vi "Maths.vi"(6 "Curseur tracé":i32, 8 "Indice curseur 2":i32, 9 "Indice curseur 1":i32, 10 "Graphe":T1(graph)) -> (0 "standard deviation":dbl caption="écart-type" format="%0.2f", 1 "valeur max":dbl, 2 "valeur min":dbl, 3 "mean":dbl caption="moyenne" format="%0.2f")   [LabVIEW 2013]
uses:
  <vilib>/Analysis/8numeric.llb/1D Numeric Integration.vi
  <vilib>/Analysis/NI_AALBase.lvlib
  <vilib>/Analysis/NI_AALPro.lvlib
panel:
  out "residue 2":dbl caption="résidu"
  out "offset":dbl
  out "damping":dbl caption="atténuation"
  out "amplitude":dbl
  out "R-square":dbl caption="R carré"
  out "residue":dbl caption="résidu"
  out "intercept":dbl caption="interception"
  out "slope":dbl caption="pente"
  out "Intégrale":dbl format="%0.4f"
  out "variance":dbl format="%0.2f"
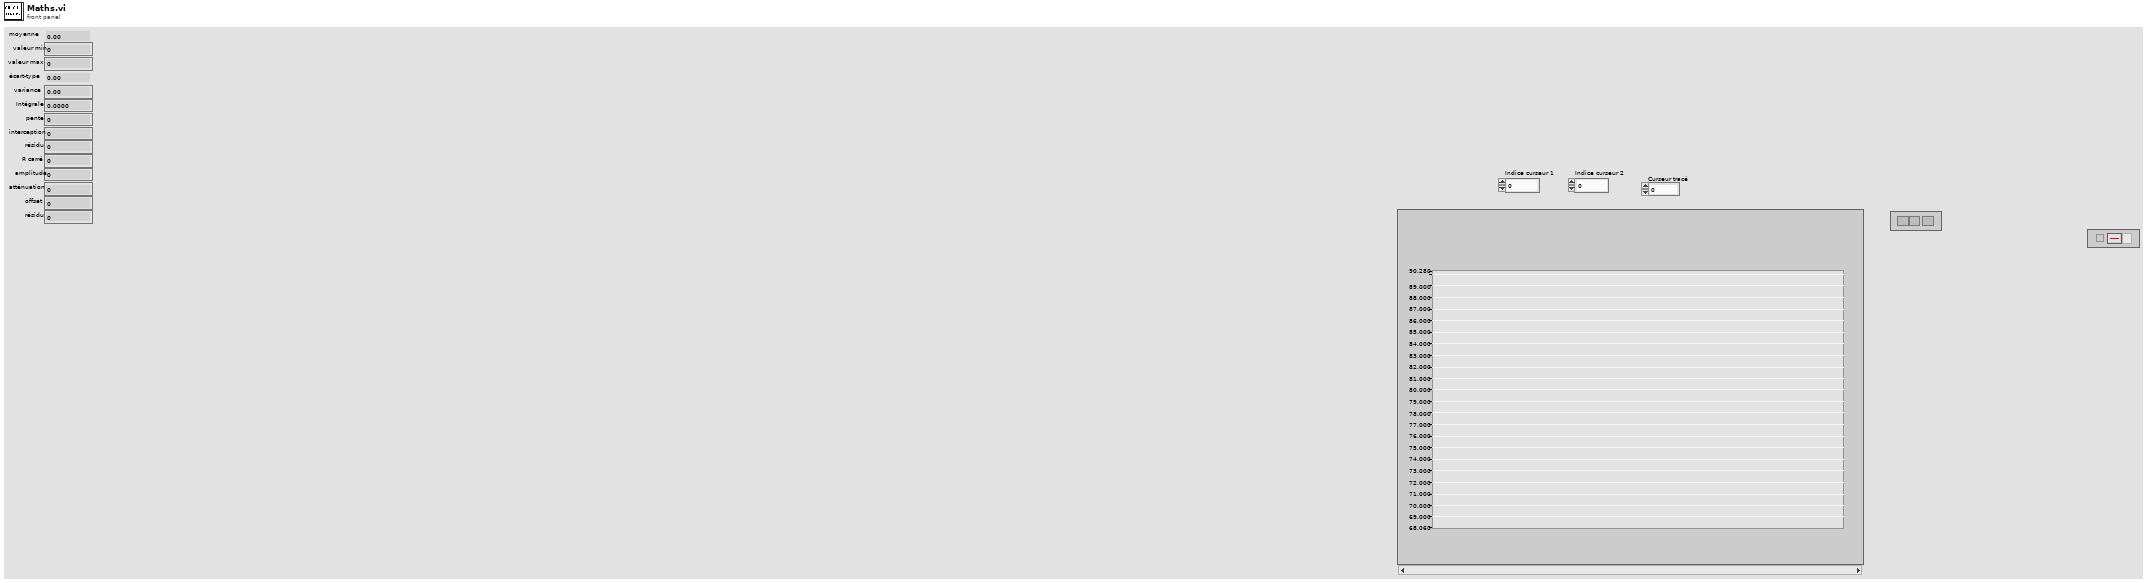
[diagram p1: front panel]
types:
  T1 = cluster{"Horodatage":timestamp[], "Donnees":dbl[]}[]
  T2 = cluster{"Horodatage":timestamp[], "Donnees":dbl[]}
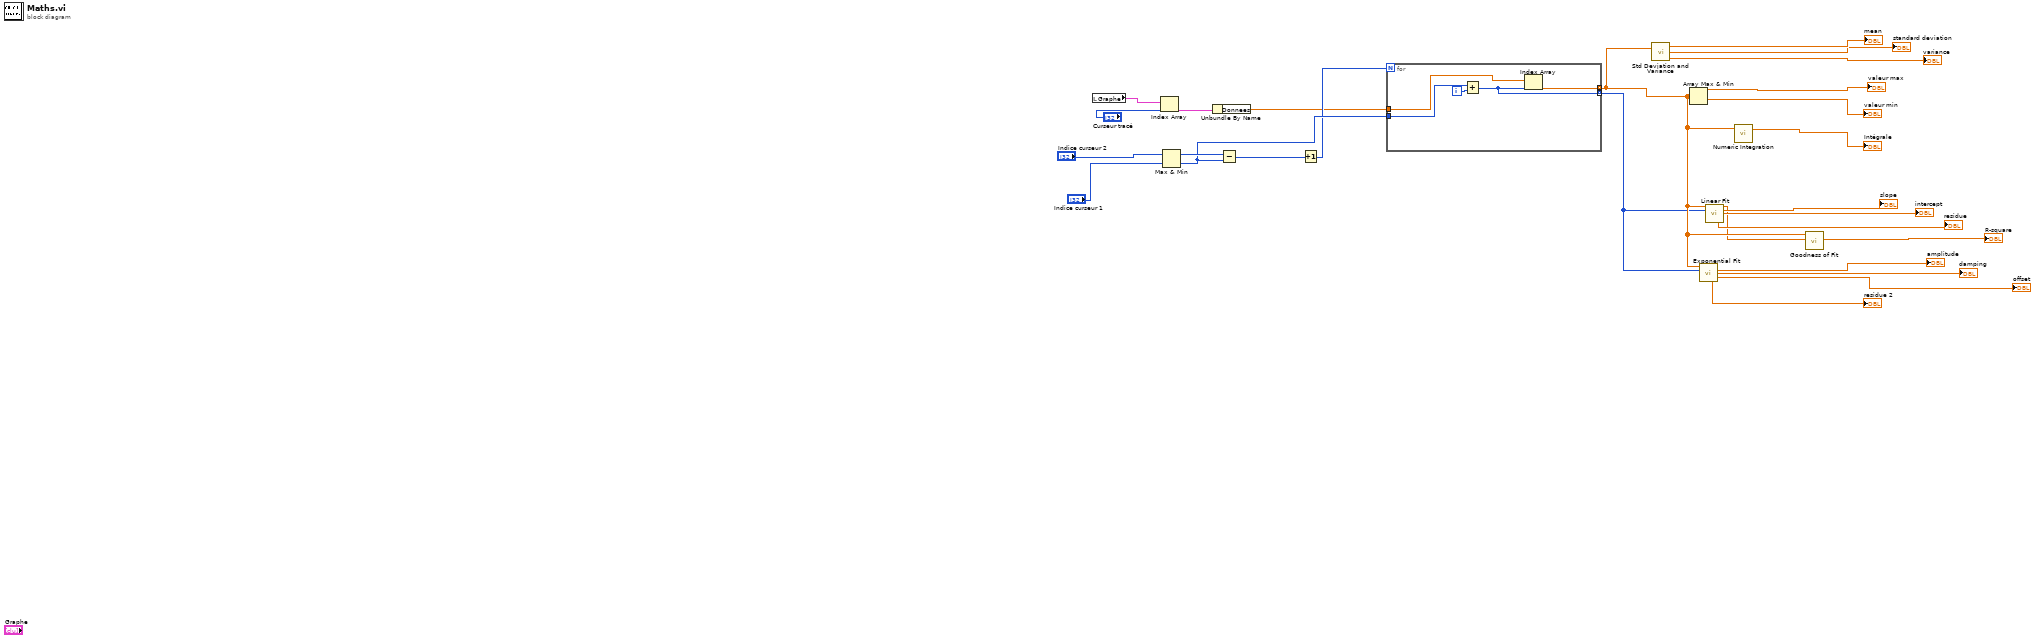
[diagram p0: block diagram]
diagram:
  n1 = local read "Graphe"() -> (w23:T1)
  n2 = Index Array(array=w23, index="Curseur tracé") -> (element=w22:T2)
  n3 = Max & Min(x="Indice curseur 2", y="Indice curseur 1") -> (max(x,y)=w27:i32, min(x,y)=w26:i32)
  n4 = Unbundle By Name(w22) -> ("Donnees"=w20:dbl[])
  n5 = Subtract(x=w27, y=w26) -> (x-y=w25:i32)
  n6 = Increment(x=w25) -> (x+1=w24:i32)
  n7 = for {
    N: w24 -> [_]
    tunnel: w26 -> [w32]
    tunnel: w20 -> [w30]
    tunnel: [w29] -> w5 mode=indexing
    tunnel: [w28] -> w2 mode=indexing
    i -> [w31]
    n8 = Add(x=w32, y=w31) -> (x+y=w28:i32)
    n9 = Index Array(array=w30, index=w28) -> (element=w29:dbl)
  }
  n10 = call <vilib>:"Std Deviation and Variance.vi"("X"=w5) -> ("mean"=→"mean":dbl, "standard deviation"=→"standard deviation":dbl, "variance"=→"variance":dbl)  [unwired: 1 in]
  n11 = Array Max & Min(array=w5) -> (max value=→"valeur max":dbl, min value=→"valeur min":dbl)  [unwired: 2 out]
  n12 = call <vilib>:"Exponential Fit.vi"("Y"=w5, "X"=w2) -> ("amplitude"=→"amplitude":dbl, "damping"=→"damping":dbl, "offset"=→"offset":dbl, "residue"=→"residue 2":dbl)  [unwired: 8 in, 2 out]
  n13 = call <vilib>:"Linear Fit.vi"("Y"=w5, "X"=w2) -> ("Best Linear Fit"=w3:dbl[], "slope"=→"slope":dbl, "intercept"=→"intercept":dbl, "residue"=→"residue":dbl)  [unwired: 9 in, 1 out]
  n14 = call-poly <vilib>:"Numeric Integration.vi"("Input Array"=w5) -> ("result"=→"Intégrale":dbl)  [unwired: 2 in, 1 out]
  n15 = call <vilib>:"Goodness of Fit.vi"("Best Fit"=w3, "Y"=w5) -> ("R-square"=→"R-square":dbl)  [unwired: 6 in, 3 out]
